vi "IRH3T(Corrected Version).vi"(8 "Due Dates":u16[](array[numeric]), 9 "Initial Tardiness":i32, 10 "Schedule 2B Improved":u16[](array[numeric]), 11 "Proocessing Times  (Machines x Jobs)":u16[][](array[numeric])=[[208, 80, 8, 184, 218, 197, 100, 5], [64, 30, 39, 91, 257, 38, 34, 447], [23, 215, 125, 135, 165, 136, 164, 37], [88, 22, 207, 5, 58, 213, 52, 355], [6, 181, 111, 222, 27, 259, 91, 103], [149, 37, 22, 14, 71, 155, 536, 16], [113, 71, 274, 348, 187, 1, 3, 3], [349, 364, 214, 1, 17, 1, 20, 34]]) -> (1 "IRH3T Schedule Out":u16[](array[numeric]), 2 "Total Tardiness":u16, 3 "IRH3T (Reordered) Schedule Out":u16[](array[numeric]))   [LabVIEW 2013]
uses:
  Classes/Scheduler_Class/Operation to Machine Job Tuple.vi
  Classes/Scheduler.lvclass
panel:
  out "String":string
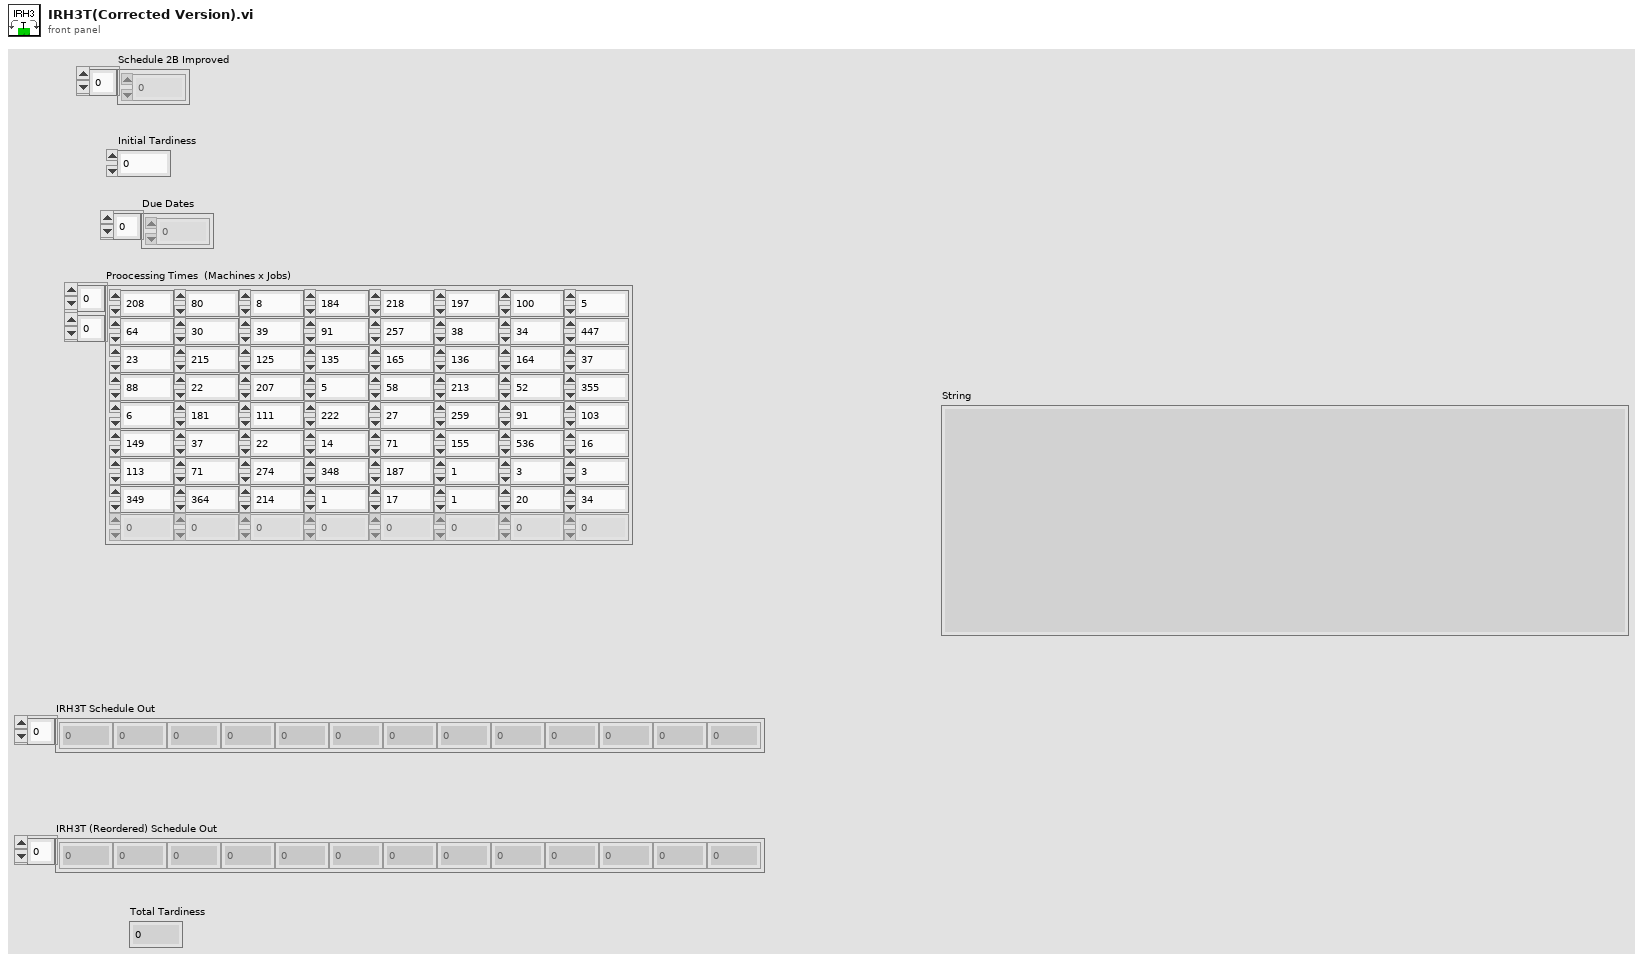
[diagram p1: front panel]
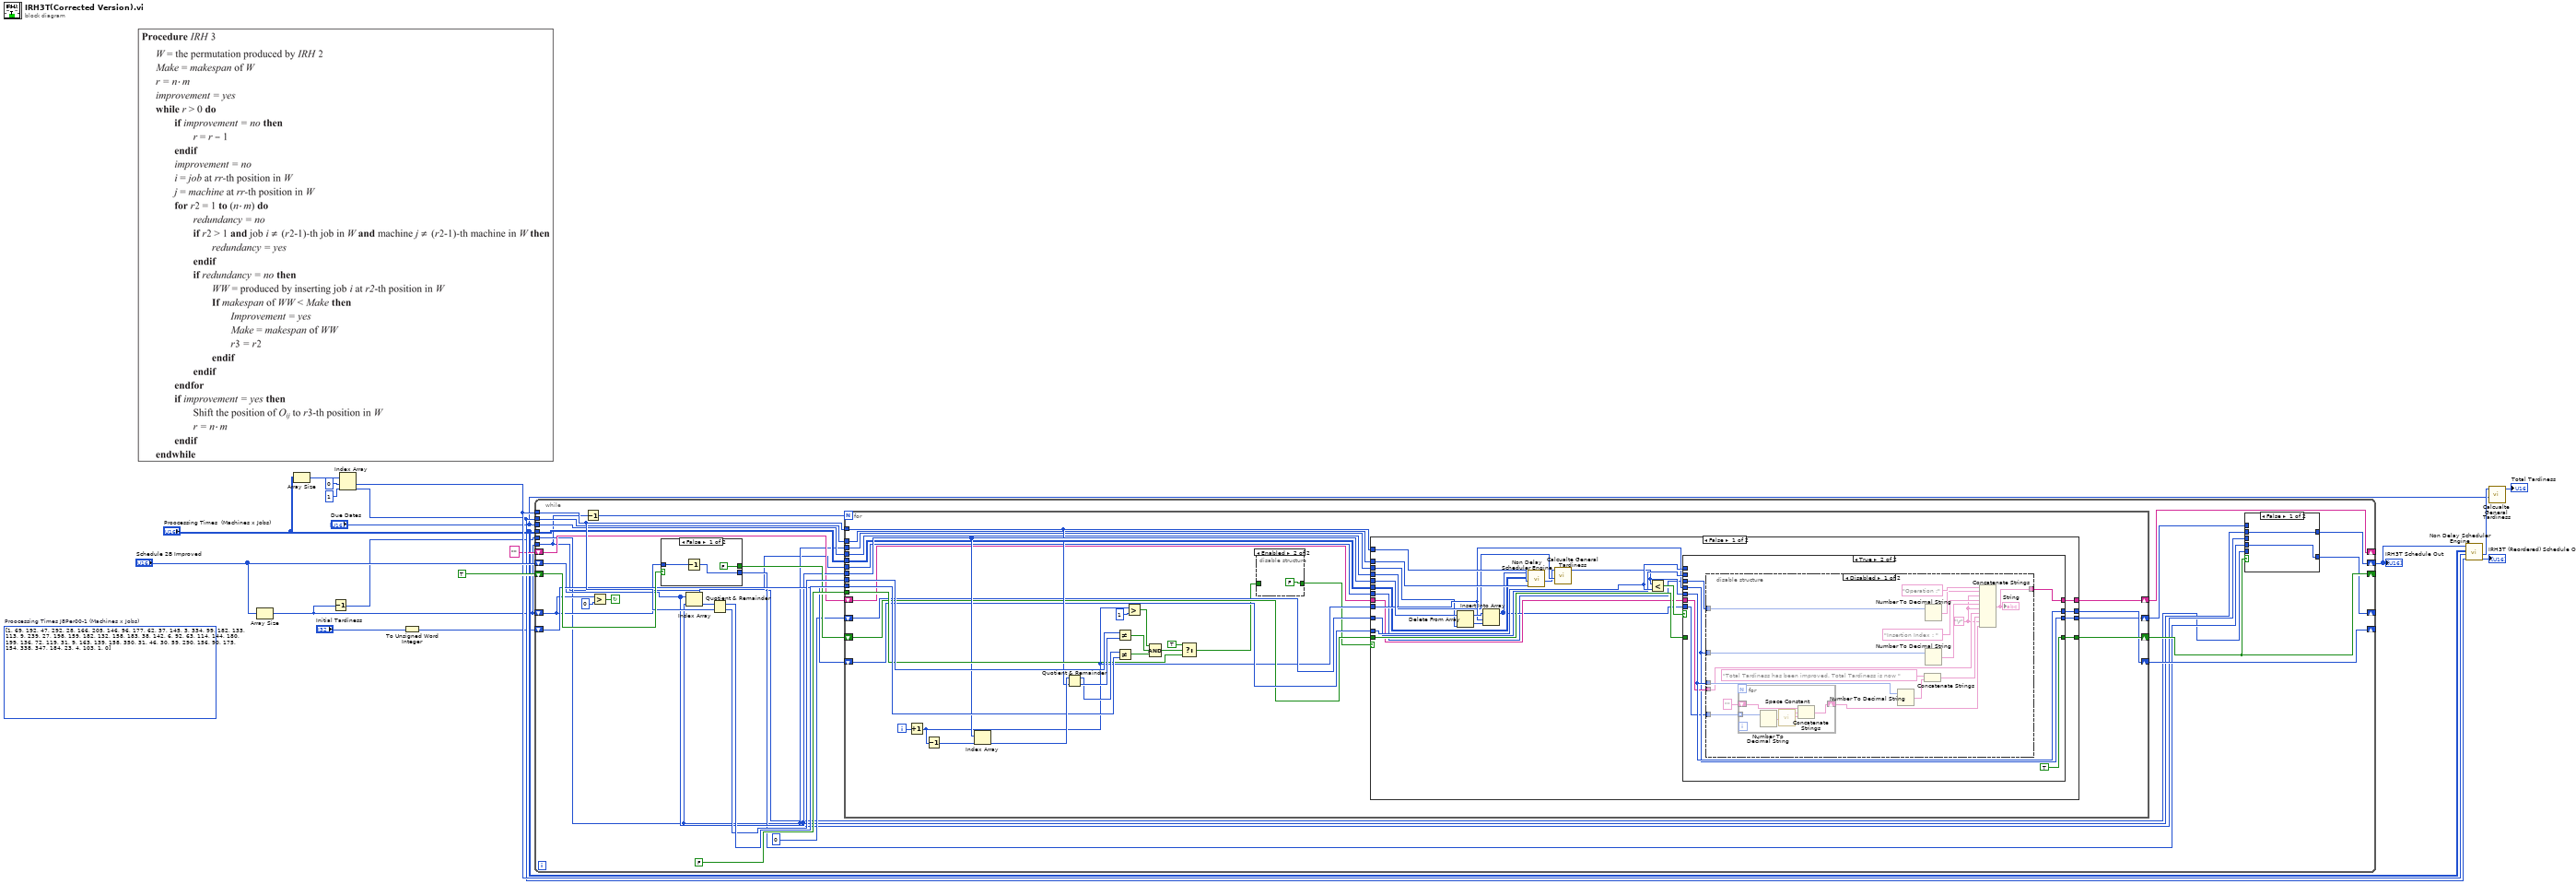
[diagram p0: block diagram]
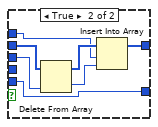
[diagram p2: hidden frame]
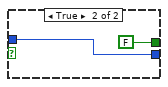
[diagram p7: hidden frame]
diagram:
  (unwired) u16[][] [[1, 69, 192, 47, 292, 28, 166, 205], [146, 96, 177, 62, 37, 145, 3, 334], [99, 182, 133, 113, 9, 239, 27, 198], [159, 182, 132, 158, 183, 38, 142, 6], [92, 63, 114, 144, 180, 199, 136, 72], [119, 31, 9, 163, 139, 158, 350, 31], [46, 30, 59, 290, 156, 90, 175, 154], [338, 347, 184, 23, 4, 103, 1, 0]]  # Proocessing Times J8Per00-1 (Machines x Jobs)
  n1 = Array Size(array="Schedule 2B Improved") -> (size(s)=w1:i32)
  n2 = Array Size(array="Proocessing Times  (Machines x Jobs)") -> (size(s)=w16:i32[])
  n3 = Decrement(x=w1) -> (x-1=w2:i32)
  n4 = Index Array(array=w16, index #1=0 ("index"), index #2=1 ("index")) -> (element #1=w12:i32, element #2=w11:i32)
  n5 = To Unsigned Word Integer(number="Initial Tardiness") -> (unsigned 16bit integer=w3:u16)
  n6 = while {
    shift-right: [w28] -> _
    shift-left: w1 -> [w26]
    shift-right: [w31] -> _
    shift-left: TRUE -> [w43]
    tunnel: w12 -> [w41]
    tunnel: "Proocessing Times  (Machines x Jobs)" -> [w38]
    tunnel: w11 -> [w37]
    tunnel: "Due Dates" -> [w36]
    shift-right: [w33] -> _
    shift-left: w3 -> [w35]
    shift-right: [w25] -> w13
    shift-left: "Schedule 2B Improved" -> [w30]
    shift-right: [w23] -> _
    shift-left: "" -> [w24]
    tunnel: w2 -> [w22]
    tunnel: w1 -> [w20]
    stop <- w44 continue-if-true
    n7 = Decrement(x=w20) -> (x-1=w19:i32)
    n8 = Greater?(x=w26, y=0) -> (0:w44:bool)
    n9 = case shown="False" w43 {
      tunnel: w26 -> [w150 w152]
      tunnel: [w149 w152] -> w27
      tunnel: [FALSE FALSE] -> w34
      frame False {
        n10 = Decrement(x=w150) -> (x-1=w149:i32)
      }
      frame True {
      }
    }
    n11 = Index Array(array=w30, index=w22) -> (element=w21:u16)
    n12 = Quotient & Remainder(x=w21, y=w41) -> (x-y*floor(x/y)=w40:i32, floor(x/y)=w39:i32)
    n13 = for {
      N: w19 -> [_]
      tunnel: FALSE -> [w77]
      tunnel: w30 -> [w75]
      tunnel: w41 -> [w73]
      tunnel: w40 -> [w80]
      tunnel: w39 -> [w84]
      tunnel: w38 -> [w74]
      tunnel: w37 -> [w72]
      tunnel: w36 -> [w71]
      shift-right: [w68] -> w31
      shift-left: w34 -> [w69]
      shift-right: [w67] -> w33
      shift-left: w35 -> [w70]
      shift-right: [w65] -> w29
      shift-left: 0 -> [w66]
      shift-right: [w63] -> w23
      shift-left: w24 -> [w64]
      tunnel: w22 -> [w58]
      tunnel: w21 -> [w57]
      i -> [w62]
      n14 = Increment(x=w62) -> (x+1=w60:i32)
      n15 = Decrement(x=w60) -> (x-1=w59:i32)
      n16 = Index Array(array=w75, index=w59) -> (element=w86:u16)
      n17 = Quotient & Remainder(x=w86, y=w73) -> (x-y*floor(x/y)=w81:i32, floor(x/y)=w83:i32)
      n18 = Not Equal?(x=w84, y=w83) -> (x != y?=w82:bool)
      n19 = Not Equal?(x=w81, y=w80) -> (x != y?=w79:bool)
      n20 = Greater?(x=w60, y=1) -> (0:w85:bool)
      n21 = Compound Arithmetic op=AND(w85, w82, w79) -> (w78:bool)
      n22 = Select(t=TRUE, s=w78, f=w77) -> (s? t:f=w56:bool)
      n23 = disable-structure shown="Enabled" {
        disable-tunnel: w56 -> [w87 _]
        disable-tunnel: [w87 FALSE ("t")] -> w55
        frame Disabled {
        }
        frame Enabled {
        }
      }
      n24 = case shown="False" w55 {
        tunnel: w75 -> [w110 _]
        tunnel: w58 -> [w92 _]
        tunnel: w60 -> [w99 _]
        tunnel: w74 -> [w96 _]
        tunnel: w73 -> [w108 _]
        tunnel: w72 -> [w107 _]
        tunnel: w71 -> [w94 _]
        tunnel: w70 -> [w102 w146]
        tunnel: w69 -> [w105 w147]
        tunnel: [w104 w147] -> w68
        tunnel: [w103 w146] -> w67
        tunnel: w66 -> [w101 w145]
        tunnel: [w100 w145] -> w65
        tunnel: w64 -> [w98 w144]
        tunnel: [w97 w144] -> w63
        tunnel: w57 -> [w89 _]
        frame False {
          n25 = Delete From Array(array=w110, index=w92) -> (deleted portion=w95:u16, array with subset deleted=w109:u16[])  [unwired: 1 in]
          n26 = Insert Into Array(array=w109, index=w99, new element=w95) -> (w90:u16[])
          n27 = call "Non Delay Scheduler Engine.vi"("Number of  Jobs"=w107, "Number of Machines"=w108, "Processing Times"=w96, "Schedule"=w90) -> ("Job Completion Times"=w91:u16[])  [unwired: 2 in, 5 out]
          n28 = call "Calcualte General Tardiness.vi"("Due Dates"=w94, "Job Completion Times"=w91) -> ("Total Tardiness (U16)"=w93:u16)  [unwired: 9 in]
          n29 = Less?(x=w93, y=w102) -> (x < y?=w106:bool)
          n30 = case shown="True" w106 {
            tunnel: [w114 TRUE] -> w104
            tunnel: w105 -> [w114 _]
            tunnel: w93 -> [_ w120]
            tunnel: [w113 w120] -> w103
            tunnel: w102 -> [w113 _]
            tunnel: w101 -> [w112 _]
            tunnel: [w112 w116] -> w100
            tunnel: w99 -> [_ w116]
            tunnel: w98 -> [w111 w119]
            tunnel: [w111 w118] -> w97
            tunnel: w90 -> [_ w115]
            tunnel: w89 -> [_ w117]
            frame False {
            }
            frame True {
              n31 = disable-structure shown="Disabled" {
                disable-tunnel: w120 -> [w137 _]
                disable-tunnel: w119 -> [w134 w143]
                disable-tunnel: [w125 w143] -> w118
                disable-tunnel: w117 -> [w132 _]
                disable-tunnel: w116 -> [w129 _]
                disable-tunnel: w115 -> [w122 _]
                frame Disabled {
                  w126 = "\r"
                  n32 = for {
                    tunnel: w122 -> [w142] mode=indexing
                    shift-right: [w138] -> w124
                    shift-left: "" -> [w141]
                    n33 = Number To Decimal String(number=w142) -> (decimal integer string=w140:string)  [unwired: 1 in]
                    n34 = call <vilib>:"Space Constant.vi"() -> ("String"=w139:string)
                    n35 = Concatenate Strings(w141, w140, w139) -> (w138:string)
                  }
                  n36 = Number To Decimal String(number=w137) -> (decimal integer string=w136:string)  [unwired: 1 in]
                  n37 = Concatenate Strings("Total Tardiness has been improved. Total Tardiness is now ", w136) -> (w133:string)
                  n38 = Number To Decimal String(number=w132) -> (decimal integer string=w130:string)  [unwired: 1 in]
                  n39 = Number To Decimal String(number=w129) -> (decimal integer string=w127:string)  [unwired: 1 in]
                  n40 = Concatenate Strings("Operation :", w130, w126, "Insertion Index : ", w127, w126, w134, w133, w126, w124) -> (w125:string)
                  "String" <- w125
                }
                frame Enabled {
                }
              }
            }
          }
        }
        frame True {
        }
      }
    }
    n41 = case shown="False" w31 {
      tunnel: w30 -> [w46 w54]
      tunnel: w29 -> [_ w52]
      tunnel: [w47 w50] -> w28
      tunnel: w20 -> [_ w50]
      tunnel: w27 -> [w47 _]
      tunnel: [w46 w49] -> w25
      tunnel: w22 -> [_ w48]
      frame False {
      }
      frame True {
        n42 = Delete From Array(array=w54, index=w48) -> (deleted portion=w51:u16, array with subset deleted=w53:u16[])  [unwired: 1 in]
        n43 = Insert Into Array(array=w53, index=w52, new element=w51) -> (w49:u16[])
      }
    }
  }
  "IRH3T Schedule Out" <- w13
  n44 = call "Non Delay Scheduler Engine.vi"("Number of  Jobs"=w11, "Number of Machines"=w12, "Processing Times"="Proocessing Times  (Machines x Jobs)", "Schedule"=w13) -> ("Reordered Schedule"=→"IRH3T (Reordered) Schedule Out":u16[], "Job Completion Times"=w7:u16[])  [unwired: 2 in, 4 out]
  n45 = call "Calcualte General Tardiness.vi"("Due Dates"="Due Dates", "Job Completion Times"=w7) -> ("Total Tardiness (U16)"=→"Total Tardiness":u16)  [unwired: 9 in]
